vi "ATF Storage-AI_V_Read.vi"(7 "number of samples per channel":i32=51, 8 "error in":errorcluster, 10 "Data FIFO Ref":T1, 11 "AI_V_Task":refnum<k21>) -> (0 "error out":errorcluster, 3 "AI_V_Task":refnum<k21>)   [LabVIEW 2022 SP3]
uses:
  RT Controls/ATF Storage-Data FIFO.ctl
  RT Controls/ATF Storage Haelth.ctl
  <vilib>/DAQmx/read.llb/DAQmx Read (Analog 1D Wfm NChan NSamp).vi
  <vilib>/DAQmx/miscellaneous.llb/DAQmx Fill In Error Info.vi
panel:
  out "overflow?":bool
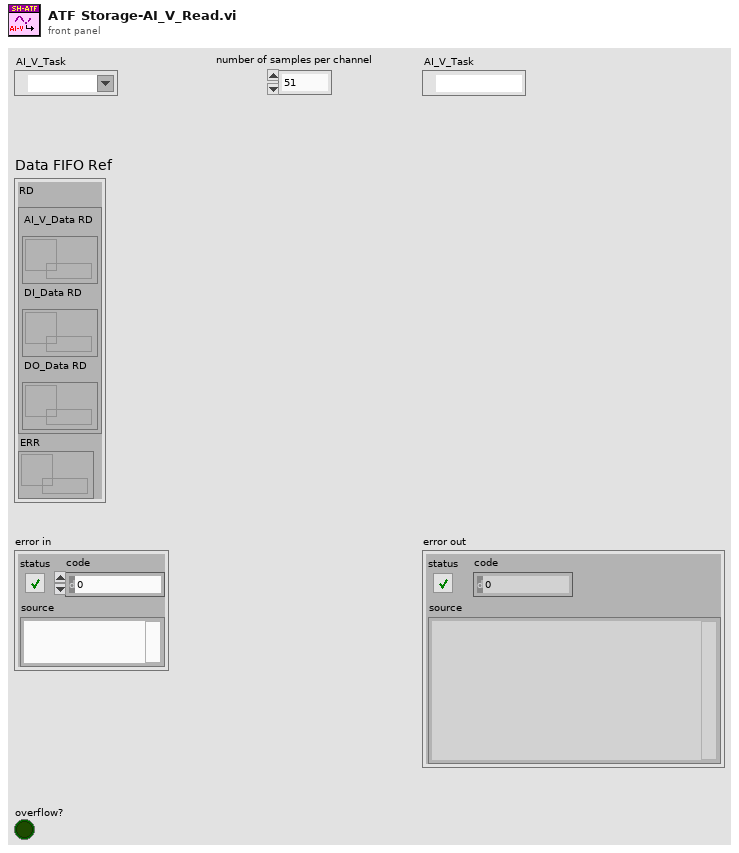
[diagram p1: front panel]
types:
  T1 = typedef "ATF Storage-Data FIFO.ctl" = cluster{"RD":cluster{"AI_V_Data RD":refnum<queue>, "DI_Data RD":refnum<queue>, "DO_Data RD":refnum<queue>}, "ERR":refnum<queue>}
  T2 = typedef "ATF Storage Haelth.ctl" = enum16{"AI C", "AI V", "AO", "DI", "DO", "TC", "ACC", "RT Str", "DR A"}
  T3 = enum16{"Init", "Read 'All'", "Read 'n'", "Read '1'", "Write '1'", "Write 'n'", "Write 'All'"}
  T4 = cluster{"Start DAQ":bool, "Stop DAQ":bool, "RT Stop":bool, "RT Exit":bool, "Start Seq":bool}
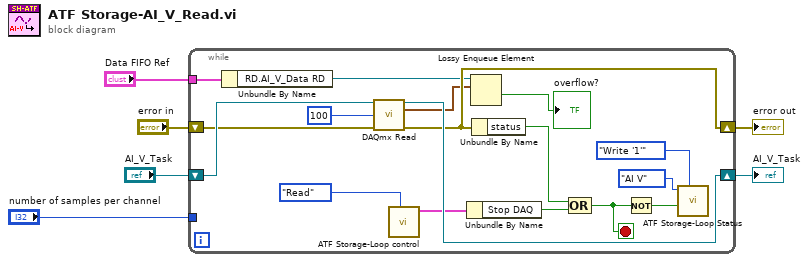
[diagram p0: block diagram]
diagram:
  n1 = while {
    shift-right: [w21] -> w1
    shift-left: "AI_V_Task" -> [w23]
    shift-right: [w20] -> w4
    shift-left: "error in" -> [w22]
    tunnel: "number of samples per channel" -> [_]
    tunnel: "Data FIFO Ref" -> [w14]
    stop <- w19 stop-if-true
    n2 = Unbundle By Name(w14) -> ("RD.AI_V_Data RD"=w11:refnum<queue>)
    n3 = call-poly <vilib>:"DAQmx Read.vi"("task/channels in"=w23, "number of samples per channel"=100, "error in"=w22) -> ("task out"=w21:refnum<k21>, "data"=w8:waveform(dbl)[], "error out"=w20:errorcluster)  [unwired: 10 in]
    n4 = call "ATF Storage-Loop control.vi"("Action"=enum16{"Init", "Write", "Read"}."Read") -> ("Loop Control out"=w17:T4)  [unwired: 9 in, 1 out]
    n5 = Unbundle By Name(w17) -> ("Stop DAQ"=w16:bool)
    n6 = Lossy Enqueue Element(queue=w11, element=w8) -> (overflow?=→"overflow?":bool)  [unwired: 1 in, 3 out]
    n7 = Unbundle By Name(w20) -> ("status"=w18:bool)
    n8 = Compound Arithmetic op=OR(w18, w16) -> (w19:bool)
    n9 = Not(x=w19) -> (.not. x?=w12:bool)
    n10 = call "ATF Storage-Loop Status.vi"("Option"=T3."Write '1'", "Status"=w12, "Loop"=ATF_Storage_Haelth."AI V") -> ()  [unwired: 6 in, 3 out]
  }
  "error out" <- w4
  "AI_V_Task" <- w1
